vi "Fc_TCP_Client_33.vi"(0 "CMD":i32(ring) items=["OCP_IF_CMD_TRACE_READ", "OCP_IF_CMD_TRACE_RESET", "OCP_IF_CMD_TRACE_GET_SIZE", "OCP_IF_CMD_TRACE_SET_SIZE", "OCP_IF_CMD_TRACE_GET_NUMBER_SIGNALS", "OCP_IF_CMD_TRACE_GET_SIGNALS_NAMES", "OCP_IF_CMD_TRACE_GET_NUMBER_TRACES", "OCP_IF_CMD_TRACE_GET_TRACES_NAMES", "OCP_IF_CMD_TRACE_GET_ADDRESS", "OCP_IF_CMD_CS_STATUS", "OCP_IF_CMD_CS_ENABLE", "OCP_IF_CMD_CS_DISABLE", "OCP_IF_CMD_CS_CONTROLLER_IF", "OCP_IF_CMD_CS_HARDWARE_IF", "OCP_IF_CMD_CS_GET_NUMBER_CONTROLLERS", "OCP_IF_CMD_CS_GET_CONTROLLERS_NAMES", "OCP_IF_CMD_PLATFORM_ID", "OCP_IF_CMD_PLATFORM_IF", "OCP_IF_CMD_OPIL_UPDATE_MEASUREMENTS", "OCP_IF_CMD_OPIL_UPDATE_SIM_DATA", "OCP_IF_CMD_OPIL_RUN_CONTROL", "OCP_IF_CMD_OPIL_INITIALIZE_CONTROL", "OCP_IF_CMD_OPIL_GET_CONTROL", "OCP_IF_CMD_OPIL_GET_CONTROLLER_DATA", "OCP_IF_CMD_END"], 2 "Input Cluster":T3, 3 "error in (no error)":errorcluster, 8 "Comunication Cluster":T1) -> (6 "Output cluster":T2, 7 "R_message 1":string, 10 "error out":errorcluster)   [LabVIEW 2022 SP3]
doc: "This function follows the tcp ip protocol to communicate with the microcontroller depending on the command (CMD) to be used. Version #33\n\nList of commands\n- 0-> OCP_IF_CMD_TRACE_READ = 0, //LV: SIZE - CMD - ID || RESPONSE: SIZE - DATA\n- 1-> OCP_IF_CMD_TRACE_RESET, //SIZE - CMD - ID || RESPONSE: SIZE\n- 2-> OCP_IF_CMD_TRACE_GET_SIZE, //SIZE - CMD - ID || RESPONSE: SIZE - TRACE_SIZE (4 bztes)\n- 3-> OCP_IF_CMD_TRACE_SET_SIZE, //SIZE - CMD - ID - TRACE_SIZE ( 4 bytes) || RESPONSE: SIZE\n- 4-> OCP_IF_CMD_TRACE_GET_NUMBER_SIGNALS, //SIZE - CMD - ID || RESPONSE: SIZE - NB_SIGNALS (4 bytes)\n- 5-> OCP_IF_CMD_TRACE_GET_SIGNALS_NAMES, //SIZE - CMD - ID || RESPONSE: SIZE - string\n- 6-> OCP_IF_CMD_TRACE_GET_NUMBER_TRACES, //SIZE - CMD || RESPONSE: SIZE - NB_TRACES (4 bytes)\n- 7-> OCP_IF_CMD_TRACE_GET_TRACES_NAMES, //SIZE - CMD || RESPONSE: SIZE - NB_TRACES (N bytes)\n- 8-> OCP_IF_CMD_TRACE_GET_ADDRESS, //SIZE - CMD - ID || RESPONSE: SIZE - TRACE ADDRESS (4 bytes)\n- 9-> OCP_IF_CMD_CS_STATUS, //SIZE - CMD - ID || RESPONSE: SIZE - CS STATUS (4 bytes)\n- 10-> OCP_IF_CMD_CS_ENABLE, //SIZE - CMD - ID || RESPONSE: SIZE\n- 11-> OCP_IF_CMD_CS_DISABLE, //SIZE - CMD - ID || RESPONSE: SIZE\n- 12-> OCP_IF_CMD_CS_CONTROLLER_IF, //SIZE - CMD - ID - DATA (N) || RESPONSE: SIZE - DATA (M)\n- 13-> OCP_IF_CMD_CS_HARDWARE_IF, //SIZE - CMD - ID - DATA (N) || RESPONSE: SIZE - DATA (M)\n- 14-> OCP_IF_CMD_CS_GET_NUMBER_CONTROLLERS, //SIZE - CMD || RESPONSE: SIZE - NB CSs\n- 15-> OCP_IF_CMD_CS_GET_CONTROLLERS_NAMES, //SIZE - CMD || RESPONSE: SIZE - string NAMES CSs"
uses:
  <vilib>/Utility/error.llb/Error Cluster From Error Code.vi
  <vilib>/ErrorRing/Error Ring.xnode
panel:
  out "R_Data string length":cluster{i32}
  out "W_Data string length: \nbytes written 2":i32
  out "W_Data string_flat":string
  # "0-> OCP_IF_CMD_TRACE_READ = 0, //LV: SIZE - CMD - ID || RESPONSE: SIZE - DATA\n1->\tOCP_IF_CMD_TRACE_RESET, //SIZE - CMD - ID || RESPONSE: SIZE\n2-> OCP_IF_CMD_TRACE_GET_SIZE, //SIZE - CMD - ID || RESPONSE: SIZE - TRACE_SIZE (4 bztes)\n3->\tOCP_IF_CMD_TRACE_SET_SIZE, //SIZE - CMD - ID - TRACE_SIZE ( 4 bytes) || RESPONSE: SIZE\n4->\tOCP_IF_CMD_TRACE_GET_NUMBER_SIGNALS, //SIZE - CMD - ID || RESPONSE: SIZE - NB_SIGNALS (4 bytes)\n5->\tOCP_IF_CMD_TRACE_GET_SIGNALS_NAMES, //SIZE - CMD - ID || RESPONSE: SIZE - string\n6->\tOCP_IF_CMD_TRACE_GET_NUMBER_TRACES, //SIZE - CMD  || RESPONSE: SIZE - NB_TRACES (4 bytes)\n7->\tOCP_IF_CMD_TRACE_GET_TRACES_NAMES, //SIZE - CMD || RESPONSE: SIZE - NB_TRACES (N bytes)\n8-> OCP_IF_CMD_TRACE_GET_ADDRESS, //SIZE - CMD - ID || RESPONSE: SIZE - TRACE ADDRESS (4 bytes)\n9-> OCP_IF_CMD_CS_STATUS, //SIZE - CMD - ID || RESPONSE: SIZE - CS STATUS (4 bytes)\n10-> OCP_IF_CMD_CS_ENABLE, //SIZE - CMD - ID || RESPONSE: SIZE\n11-> OCP_IF_CMD_CS_DISABLE, //SIZE - CMD - ID || RESPONSE: SIZE\n12-> OCP_IF_CMD_CS_CONTROLLER_IF, //SIZE - CMD - ID - DATA (N) || RESPONSE: SIZE - DATA (M)\n13-> OCP_IF_CMD_CS_HARDWARE_IF, //SIZE - CMD - ID - DATA (N) || RESPONSE: SIZE - DATA (M)\n14-> OCP_IF_CMD_CS_GET_NUMBER_CONTROLLERS, //SIZE - CMD || RESPONSE: SIZE - NB CSs\n15-> OCP_IF_CMD_CS_GET_CONTROLLERS_NAMES, //SIZE - CMD || RESPONSE: SIZE - string NAMES CSs"
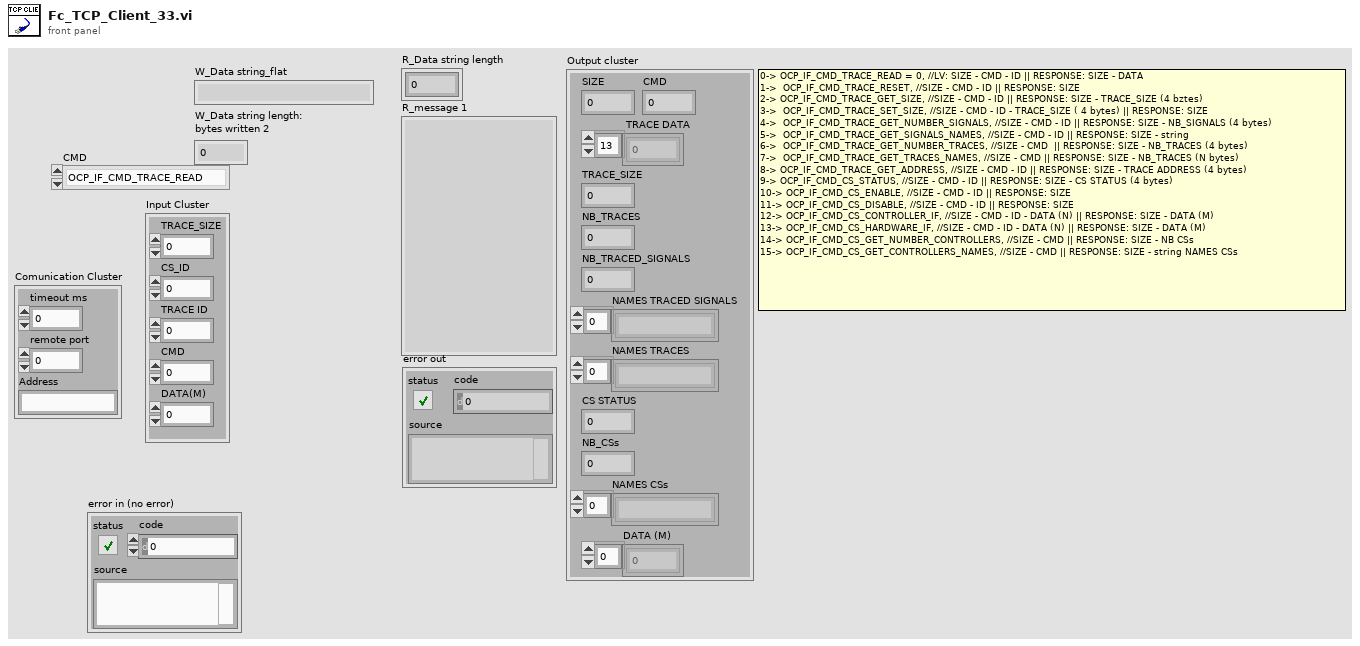
[diagram p1: front panel]
types:
  T1 = cluster{"timeout ms":i32, "remote port":u16, "Address":string}
  T2 = cluster{"SIZE":i32, " TRACE DATA":sgl[], "TRACE_SIZE":i32, "NB_TRACES":i32, "NB_TRACED_SIGNALS":i32, "NAMES TRACED SIGNALS":string[], "NAMES TRACES":string[], "CS STATUS":i32, "NB_CSs":i32, "NAMES CSs":string[], "DATA (M)":sgl[], "CMD":i32}
  T3 = cluster{"TRACE_SIZE":i32, "CS_ID":i32, "TRACE ID":i32, "CMD":i32, "DATA(M)":i32}
  T4 = enum16{"big-endian, network order", "native, host order", "little-endian"}
  T5 = enum16{"Standard", "Buffered", "CRLF", "Immediate"}
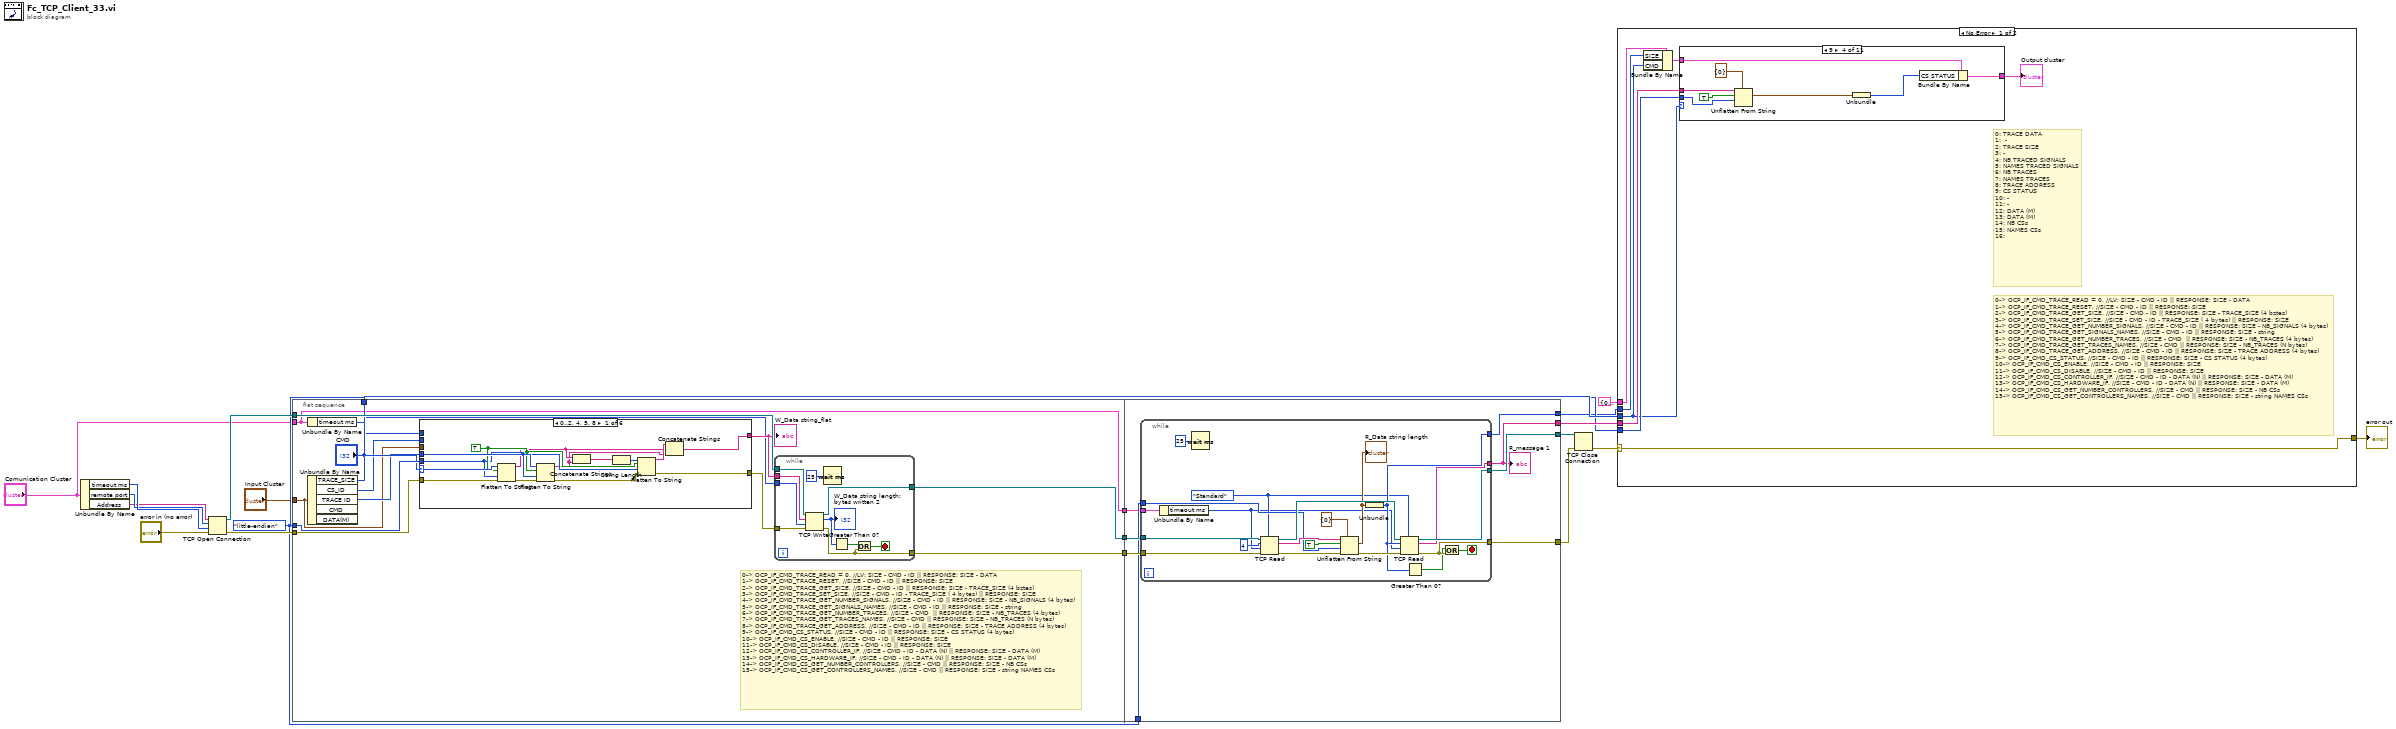
[diagram p0: block diagram]
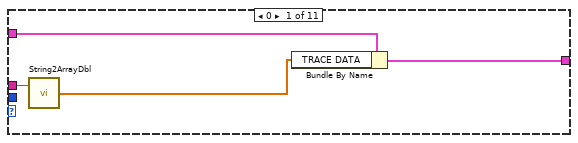
[diagram p2: hidden frame]
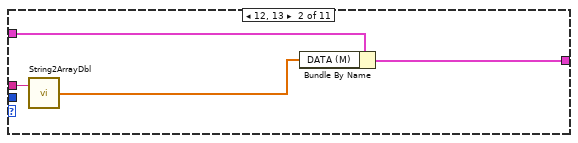
[diagram p3: hidden frame]
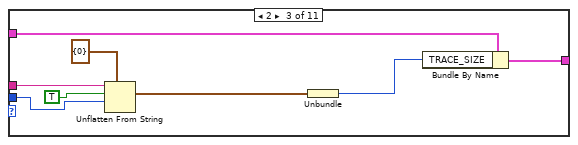
[diagram p4: hidden frame]
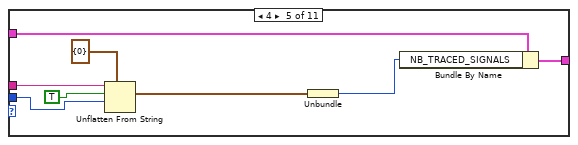
[diagram p5: hidden frame]
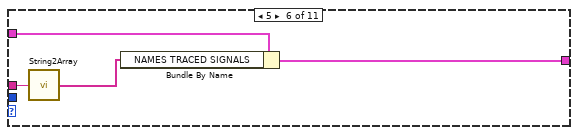
[diagram p6: hidden frame]
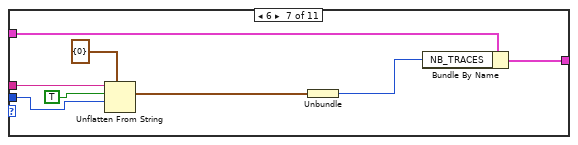
[diagram p7: hidden frame]
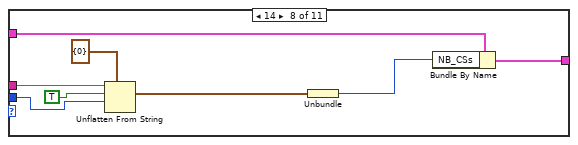
[diagram p8: hidden frame]
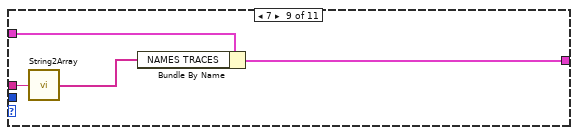
[diagram p9: hidden frame]
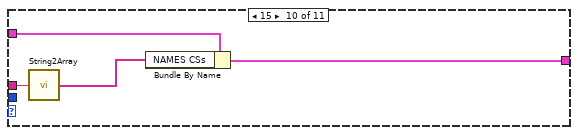
[diagram p10: hidden frame]
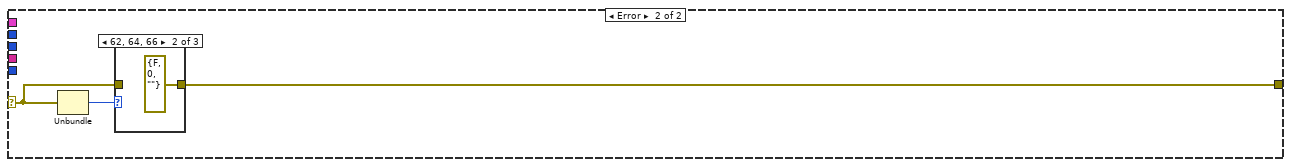
[diagram p12: hidden frame]
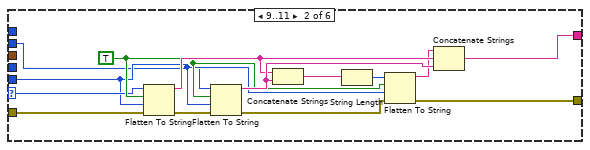
[diagram p15: hidden frame]
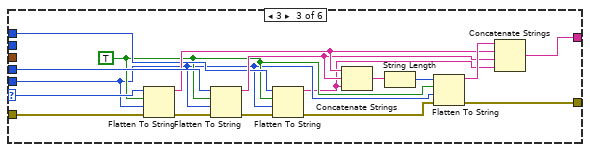
[diagram p16: hidden frame]
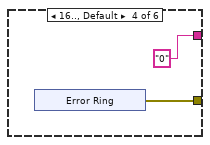
[diagram p17: hidden frame]
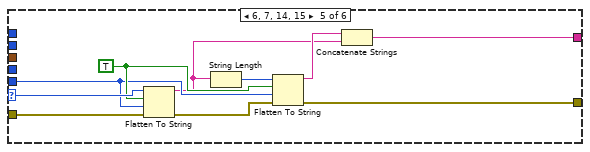
[diagram p18: hidden frame]
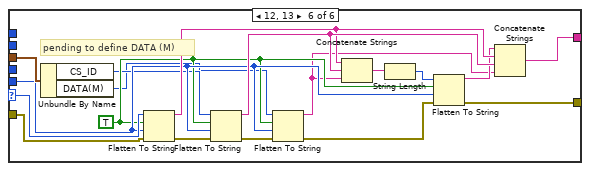
[diagram p19: hidden frame]
diagram:
  w8 = T4."little-endian" ("byte order (0:big-endian, network order)")
  n1 = Unbundle By Name("Comunication Cluster") -> ("timeout ms"=w4:i32, "remote port"=w3:u16, "Address"=w2:string)
  n2 = TCP Open Connection(address=w2, remote port or service name=w3, timeout ms (60000)=w4, error in (no error)="error in (no error)") -> (connection ID=w20:refnum<k5>, error out=w19:errorcluster)  [unwired: 1 in]
  n3 = flat-sequence {
    tunnel: w20 -> [w34]
    tunnel: w19 -> [w31]
    tunnel: [w33] -> w18
    tunnel: [w32] -> w17
    tunnel: w8 -> [w30]
    tunnel: ["CMD"] -> w11
    tunnel: "Input Cluster" -> [w24]
    tunnel: "Comunication Cluster" -> [w22]
    tunnel: [w22] -> w1
    tunnel: w18 -> [w132]
    tunnel: w17 -> [w131]
    tunnel: [w130] -> w14
    tunnel: [w129] -> w13
    tunnel: w8 -> [w128]
    tunnel: [w127] -> w10
    tunnel: [w126] -> w7
    tunnel: w1 -> [w125]
    frame #0 {
      # "0-> OCP_IF_CMD_TRACE_READ = 0, //LV: SIZE - CMD - ID || RESPONSE: SIZE - DATA\n1->\tOCP_IF_CMD_TRACE_RESET, //SIZE - CMD - ID || RESPONSE: SIZE\n2-> OCP_IF_CMD_TRACE_GET_SIZE, //SIZE - CMD - ID || RESPONSE: SIZE - TRACE_SIZE (4 bztes)\n3->\tOCP_IF_CMD_TRACE_SET_SIZE, //SIZE - CMD - ID - TRACE_SIZE ( 4 bytes) || RESPONSE: SIZE\n4->\tOCP_IF_CMD_TRACE_GET_NUMBER_SIGNALS, //SIZE - CMD - ID || RESPONSE: SIZE - NB_SIGNALS (4 bytes)\n5->\tOCP_IF_CMD_TRACE_GET_SIGNALS_NAMES, //SIZE - CMD - ID || RESPONSE: SIZE - string\n6->\tOCP_IF_CMD_TRACE_GET_NUMBER_TRACES, //SIZE - CMD  || RESPONSE: SIZE - NB_TRACES (4 bytes)\n7->\tOCP_IF_CMD_TRACE_GET_TRACES_NAMES, //SIZE - CMD || RESPONSE: SIZE - NB_TRACES (N bytes)\n8-> OCP_IF_CMD_TRACE_GET_ADDRESS, //SIZE - CMD - ID || RESPONSE: SIZE - TRACE ADDRESS (4 bytes)\n9-> OCP_IF_CMD_CS_STATUS, //SIZE - CMD - ID || RESPONSE: SIZE - CS STATUS (4 bytes)\n10-> OCP_IF_CMD_CS_ENABLE, //SIZE - CMD - ID || RESPONSE: SIZE\n11-> OCP_IF_CMD_CS_DISABLE, //SIZE - CMD - ID || RESPONSE: SIZE\n12-> OCP_IF_CMD_CS_CONTROLLER_IF, //SIZE - CMD - ID - DATA (N) || RESPONSE: SIZE - DATA (M)\n13-> OCP_IF_CMD_CS_HARDWARE_IF, //SIZE - CMD - ID - DATA (N) || RESPONSE: SIZE - DATA (M)\n14-> OCP_IF_CMD_CS_GET_NUMBER_CONTROLLERS, //SIZE - CMD || RESPONSE: SIZE - NB CSs\n15-> OCP_IF_CMD_CS_GET_CONTROLLERS_NAMES, //SIZE - CMD || RESPONSE: SIZE - string NAMES CSs"
      n4 = Unbundle By Name(w24) -> ("TRACE_SIZE"=w25:i32, "CS_ID"=w27:i32, "TRACE ID"=w26:i32)  [unwired: 2 out]
      n5 = Unbundle By Name(w22) -> ("timeout ms"=w23:i32)
      n6 = case shown="0..2, 4, 5, 8" "CMD" {
        selector: "CMD" -> [w56 w63 w87 _ w105 w116]
        tunnel: w31 -> [w58 w64 w89 _ w106 w115]
        tunnel: w30 -> [w49 w62 w75 _ w101 w112]
        tunnel: w26 -> [w55 _ w86 _ _ _]
        tunnel: [w48 w60 w82 "0" w100 w118] -> w29
        tunnel: [w47 w59 w74 w91 w98 w117] -> w21
        tunnel: w25 -> [_ _ w77 _ _ _]
        tunnel: w27 -> [_ w61 _ _ _ _]
        tunnel: w24 -> [_ _ _ _ _ w114]
        frame 0..2, 4, 5, 8 {
          w50 = TRUE ("prepend array or string size? (T)")
          n7 = Flatten To String(anything=w56, prepend array or string size? (T)=w50, byte order (0:big-endian, network order)=w49, error in (no error)=w58) -> (data string=w46:string, error out=w57:errorcluster)  [unwired: 1 out]
          n8 = Flatten To String(anything=w55, prepend array or string size? (T)=w50, byte order (0:big-endian, network order)=w49, error in (no error)=w57) -> (data string=w45:string, error out=w52:errorcluster)  [unwired: 1 out]
          n9 = Concatenate Strings(w46, w45) -> (w54:string)
          n10 = String Length(string=w54) -> (length=w53:i32)
          n11 = Flatten To String(anything=w53, prepend array or string size? (T)=w50, byte order (0:big-endian, network order)=w49, error in (no error)=w52) -> (data string=w51:string, error out=w47:errorcluster)  [unwired: 1 out]
          n12 = Concatenate Strings(w51, w46, w45) -> (w48:string)
        }
        frame 9..11 {
          w65 = TRUE ("prepend array or string size? (T)")
          n13 = Flatten To String(anything=w63, prepend array or string size? (T)=w65, byte order (0:big-endian, network order)=w62, error in (no error)=w64) -> (data string=w71:string, error out=w66:errorcluster)  [unwired: 1 out]
          n14 = Flatten To String(anything=w61, prepend array or string size? (T)=w65, byte order (0:big-endian, network order)=w62, error in (no error)=w66) -> (data string=w72:string, error out=w69:errorcluster)  [unwired: 1 out]
          n15 = Concatenate Strings(w71, w72) -> (w67:string)
          n16 = String Length(string=w67) -> (length=w68:i32)
          n17 = Flatten To String(anything=w68, prepend array or string size? (T)=w65, byte order (0:big-endian, network order)=w62, error in (no error)=w69) -> (data string=w70:string, error out=w59:errorcluster)  [unwired: 1 out]
          n18 = Concatenate Strings(w70, w71, w72) -> (w60:string)
        }
        frame 3 {
          w76 = TRUE ("prepend array or string size? (T)")
          n19 = Flatten To String(anything=w87, prepend array or string size? (T)=w76, byte order (0:big-endian, network order)=w75, error in (no error)=w89) -> (data string=w81:string, error out=w88:errorcluster)  [unwired: 1 out]
          n20 = Flatten To String(anything=w86, prepend array or string size? (T)=w76, byte order (0:big-endian, network order)=w75, error in (no error)=w88) -> (data string=w80:string, error out=w79:errorcluster)  [unwired: 1 out]
          n21 = Flatten To String(anything=w77, prepend array or string size? (T)=w76, byte order (0:big-endian, network order)=w75, error in (no error)=w79) -> (data string=w73:string, error out=w78:errorcluster)  [unwired: 1 out]
          n22 = Concatenate Strings(w81, w80, w73) -> (w85:string)
          n23 = String Length(string=w85) -> (length=w84:i32)
          n24 = Flatten To String(anything=w84, prepend array or string size? (T)=w76, byte order (0:big-endian, network order)=w75, error in (no error)=w78) -> (data string=w83:string, error out=w74:errorcluster)  [unwired: 1 out]
          n25 = Concatenate Strings(w83, w81, w80, w73) -> (w82:string)
        }
        frame 16.., Default {
          n26 = xnode "Error Ring"() -> ("error out"=w91:errorcluster)
        }
        frame 6, 7, 14, 15 {
          w102 = TRUE ("prepend array or string size? (T)")
          n27 = Flatten To String(anything=w105, prepend array or string size? (T)=w102, byte order (0:big-endian, network order)=w101, error in (no error)=w106) -> (data string=w97:string, error out=w99:errorcluster)  [unwired: 1 out]
          n28 = String Length(string=w97) -> (length=w104:i32)
          n29 = Flatten To String(anything=w104, prepend array or string size? (T)=w102, byte order (0:big-endian, network order)=w101, error in (no error)=w99) -> (data string=w103:string, error out=w98:errorcluster)  [unwired: 1 out]
          n30 = Concatenate Strings(w103, w97) -> (w100:string)
        }
        frame 12, 13 {
          w111 = TRUE ("prepend array or string size? (T)")
          # "pending to define DATA (M)"
          n31 = Unbundle By Name(w114) -> ("CS_ID"=w110:i32, "DATA(M)"=w109:i32)
          n32 = Flatten To String(anything=w116, prepend array or string size? (T)=w111, byte order (0:big-endian, network order)=w112, error in (no error)=w115) -> (data string=w123:string, error out=w119:errorcluster)  [unwired: 1 out]
          n33 = Flatten To String(anything=w110, prepend array or string size? (T)=w111, byte order (0:big-endian, network order)=w112, error in (no error)=w119) -> (data string=w124:string, error out=w113:errorcluster)  [unwired: 1 out]
          n34 = Flatten To String(anything=w109, prepend array or string size? (T)=w111, byte order (0:big-endian, network order)=w112, error in (no error)=w113) -> (data string=w108:string, error out=w107:errorcluster)  [unwired: 1 out]
          n35 = Concatenate Strings(w123, w124, w108) -> (w120:string)
          n36 = String Length(string=w120) -> (length=w121:i32)
          n37 = Flatten To String(anything=w121, prepend array or string size? (T)=w111, byte order (0:big-endian, network order)=w112, error in (no error)=w107) -> (data string=w122:string, error out=w117:errorcluster)  [unwired: 1 out]
          n38 = Concatenate Strings(w122, w123, w124, w108) -> (w118:string)
        }
      }
      "W_Data string_flat" <- w29
      n39 = while {
        tunnel: w29 -> [w42]
        tunnel: w23 -> [w41]
        tunnel: w21 -> [w40]
        tunnel: [w38] -> w33
        tunnel: w34 -> [w44]
        tunnel: [w43] -> w32
        stop <- w39 stop-if-true
        n40 = TCP Write(connection ID=w44, data in=w42, error in (no error)=w40, 9:w41) -> (connection ID out=w43:refnum<k5>, bytes written=w37:i32, error out=w38:errorcluster)
        "W_Data string length: \nbytes written 2" <- w37
        n41 = Wait (ms)(milliseconds to wait=u32 25) -> ()  [unwired: 1 out]
        n42 = Greater Than 0?(x=w37) -> (x > 0?=w36:bool)
        n43 = Or(x=w36, y=w38) -> (x .or. y?=w39:bool)
      }
    }
    frame #1 {
      n44 = while {
        tunnel: w128 -> [w143]
        tunnel: [w141] -> w127
        tunnel: [w138] -> w126
        tunnel: w131 -> [w151]
        tunnel: [w150] -> w130
        tunnel: w132 -> [w152]
        tunnel: [w140] -> w129
        tunnel: w125 -> [w134]
        stop <- w139 stop-if-true
        w136 = T5."Standard" ("mode (standard)")
        n45 = Unbundle By Name(w134) -> ("timeout ms"=w135:i32)
        n46 = Wait (ms)(milliseconds to wait=u32 25) -> ()  [unwired: 1 out]
        n47 = TCP Read(connection ID=w151, bytes to read=4, error in (no error)=w152, 7:w136, 9:w135) -> (connection ID out=w153:refnum<k5>, data out=w149:string, error out=w145:errorcluster)
        n48 = Unflatten From String(type=cluster{i32} {0}, binary string=w149, data includes array or string size? (T)=TRUE, byte order (0:big-endian, network order)=w143, error in (no error)=w145) -> (value=w146:cluster{i32}, error out=w144:errorcluster)  [unwired: 1 out]
        "R_Data string length" <- w146
        n49 = Unbundle(w146) -> (w138:i32)
        n50 = TCP Read(connection ID=w153, bytes to read=w138, error in (no error)=w144, 7:w136, 9:w135) -> (connection ID out=w150:refnum<k5>, data out=w141:string, error out=w140:errorcluster)
        n51 = Greater Than 0?(x=w138) -> (x > 0?=w137:bool)
        n52 = Or(x=w137, y=w140) -> (x .or. y?=w139:bool)
      }
      "R_message 1" <- w127
    }
  }
  n53 = TCP Close Connection(connection ID=w14, error in (no error)=w13) -> (error out=w15:errorcluster)  [unwired: 1 in, 1 out]
  n54 = case shown="No Error" w15 {
    selector: w15 -> [w161 w224]
    tunnel: [w161 w223] -> w16
    tunnel: w11 -> [w155 _]
    tunnel: w10 -> [w157 _]
    tunnel: T2 {"SIZE"=0, " TRACE DATA"=[], "TRACE_SIZE"=0, "NB_TRACES"=0, "NB_TRACED_SIGNALS"=0, "NAMES TRACED SIGNALS"=[], "NAMES TRACES"=[], "CS STATUS"=0, "NB_CSs"=0, "NAMES CSs"=[], "DATA (M)"=[], "CMD"=0} ("input cluster") -> [w160 _]
    tunnel: w8 -> [w156 _]
    tunnel: w7 -> [w158 _]
    frame No Error {
      # "0: TRACE DATA\n1:  -\n2: TRACE SIZE\n3: -\n4: NB TRACED SIGNALS\n5: NAMES TRACED SIGNALS\n6: NB TRACES\n7: NAMES TRACES\n8: TRACE ADDRESS\n9: CS STATUS\n10: -\n11: -\n12: DATA (M)\n13: DATA (M)\n14: NB CSs \n15: NAMES CSs \n16:"
      # "0-> OCP_IF_CMD_TRACE_READ = 0, //LV: SIZE - CMD - ID || RESPONSE: SIZE - DATA\n1->\tOCP_IF_CMD_TRACE_RESET, //SIZE - CMD - ID || RESPONSE: SIZE\n2-> OCP_IF_CMD_TRACE_GET_SIZE, //SIZE - CMD - ID || RESPONSE: SIZE - TRACE_SIZE (4 bztes)\n3->\tOCP_IF_CMD_TRACE_SET_SIZE, //SIZE - CMD - ID - TRACE_SIZE ( 4 bytes) || RESPONSE: SIZE\n4->\tOCP_IF_CMD_TRACE_GET_NUMBER_SIGNALS, //SIZE - CMD - ID || RESPONSE: SIZE - NB_SIGNALS (4 bytes)\n5->\tOCP_IF_CMD_TRACE_GET_SIGNALS_NAMES, //SIZE - CMD - ID || RESPONSE: SIZE - string\n6->\tOCP_IF_CMD_TRACE_GET_NUMBER_TRACES, //SIZE - CMD  || RESPONSE: SIZE - NB_TRACES (4 bytes)\n7->\tOCP_IF_CMD_TRACE_GET_TRACES_NAMES, //SIZE - CMD || RESPONSE: SIZE - NB_TRACES (N bytes)\n8-> OCP_IF_CMD_TRACE_GET_ADDRESS, //SIZE - CMD - ID || RESPONSE: SIZE - TRACE ADDRESS (4 bytes)\n9-> OCP_IF_CMD_CS_STATUS, //SIZE - CMD - ID || RESPONSE: SIZE - CS STATUS (4 bytes)\n10-> OCP_IF_CMD_CS_ENABLE, //SIZE - CMD - ID || RESPONSE: SIZE\n11-> OCP_IF_CMD_CS_DISABLE, //SIZE - CMD - ID || RESPONSE: SIZE\n12-> OCP_IF_CMD_CS_CONTROLLER_IF, //SIZE - CMD - ID - DATA (N) || RESPONSE: SIZE - DATA (M)\n13-> OCP_IF_CMD_CS_HARDWARE_IF, //SIZE - CMD - ID - DATA (N) || RESPONSE: SIZE - DATA (M)\n14-> OCP_IF_CMD_CS_GET_NUMBER_CONTROLLERS, //SIZE - CMD || RESPONSE: SIZE - NB CSs\n15-> OCP_IF_CMD_CS_GET_CONTROLLERS_NAMES, //SIZE - CMD || RESPONSE: SIZE - string NAMES CSs"
      n55 = Bundle By Name(cluster=w160, "SIZE"=w158, "CMD"=w155) -> (w159:T2)
      n56 = case shown="9" w155 {
        tunnel: [w164 w168 w176 w184 w192 w196 w205 w213 w216 w220 w222] -> w154
        tunnel: w159 -> [w165 w169 w177 w185 w193 w197 w202 w210 w217 w221 w222]
        tunnel: w157 -> [w162 w166 w174 w182 w189 w195 w200 w208 w215 w219 _]
        tunnel: w156 -> [_ _ w172 w180 w188 _ w201 w209 _ _ _]
        frame 0 {
          n57 = call "String2ArrayDbl.vi"("R_message 1"=w162) -> ("Array"=w163:sgl[])  [unwired: 1 in]
          n58 = Bundle By Name(cluster=w165, "TRACE DATA"=w163) -> (w164:T2)
        }
        frame 12, 13 {
          n59 = call "String2ArrayDbl.vi"("R_message 1"=w166) -> ("Array"=w167:sgl[])  [unwired: 1 in]
          n60 = Bundle By Name(cluster=w169, "DATA (M)"=w167) -> (w168:T2)
        }
        frame 2 {
          n61 = Unflatten From String(type=cluster{i32} {0}, binary string=w174, data includes array or string size? (T)=TRUE, byte order (0:big-endian, network order)=w172) -> (value=w171:cluster{i32})  [unwired: 1 in, 2 out]
          n62 = Unbundle(w171) -> (w170:i32)
          n63 = Bundle By Name(cluster=w177, "TRACE_SIZE"=w170) -> (w176:T2)
        }
        frame 9 {
          n64 = Unflatten From String(type=cluster{i32} {0}, binary string=w182, data includes array or string size? (T)=TRUE, byte order (0:big-endian, network order)=w180) -> (value=w179:cluster{i32})  [unwired: 1 in, 2 out]
          n65 = Unbundle(w179) -> (w178:i32)
          n66 = Bundle By Name(cluster=w185, "CS STATUS"=w178) -> (w184:T2)
        }
        frame 4 {
          n67 = Unflatten From String(type=cluster{i32} {0}, binary string=w189, data includes array or string size? (T)=TRUE, byte order (0:big-endian, network order)=w188) -> (value=w190:cluster{i32})  [unwired: 1 in, 2 out]
          n68 = Unbundle(w190) -> (w186:i32)
          n69 = Bundle By Name(cluster=w193, "NB_TRACED_SIGNALS"=w186) -> (w192:T2)
        }
        frame 5 {
          n70 = call "String2Array.vi"("R_message 1"=w195) -> ("Array 2"=w194:string[])
          n71 = Bundle By Name(cluster=w197, "NAMES TRACED SIGNALS"=w194) -> (w196:T2)
        }
        frame 6 {
          n72 = Unflatten From String(type=cluster{i32} {0}, binary string=w200, data includes array or string size? (T)=TRUE, byte order (0:big-endian, network order)=w201) -> (value=w204:cluster{i32})  [unwired: 1 in, 2 out]
          n73 = Unbundle(w204) -> (w198:i32)
          n74 = Bundle By Name(cluster=w202, "NB_TRACES"=w198) -> (w205:T2)
        }
        frame 14 {
          n75 = Unflatten From String(type=cluster{i32} {0}, binary string=w208, data includes array or string size? (T)=TRUE, byte order (0:big-endian, network order)=w209) -> (value=w212:cluster{i32})  [unwired: 1 in, 2 out]
          n76 = Unbundle(w212) -> (w206:i32)
          n77 = Bundle By Name(cluster=w210, "NB_CSs"=w206) -> (w213:T2)
        }
        frame 7 {
          n78 = call "String2Array.vi"("R_message 1"=w215) -> ("Array 2"=w214:string[])
          n79 = Bundle By Name(cluster=w217, "NAMES TRACES"=w214) -> (w216:T2)
        }
        frame 15 {
          n80 = call "String2Array.vi"("R_message 1"=w219) -> ("Array 2"=w218:string[])
          n81 = Bundle By Name(cluster=w221, "NAMES CSs"=w218) -> (w220:T2)
        }
        frame 8, Default {
        }
      }
      "Output cluster" <- w154
    }
    frame Error {
      n82 = Unbundle(w224) -> ("code"=w225:i32)  [unwired: 2 out]
      n83 = case shown="62, 64, 66" w225 {
        tunnel: [w226 errorcluster {"status"=FALSE, "code"=0, "source"=""} ("error IO") w228] -> w223
        tunnel: w224 -> [w226 _ w228]
        frame 0, Default {
        }
        frame 62, 64, 66 {
        }
        frame 56 {
        }
      }
    }
  }
  "error out" <- w16
